vi "PipBoy_ReadFileConf.vi"(8 "error in (no error)":errorcluster) -> (0 "error out":errorcluster, 2 "FileConf":T1)   [LabVIEW 2014]
uses:
  ctls/PipBoy_FileConf.ctl
  <vilib>/Utility/config.llb/NI_LVConfig.lvlib
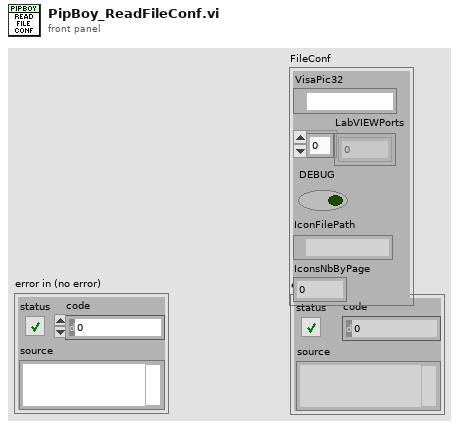
[diagram p1: front panel]
types:
  T1 = typedef "PipBoy_FileConf.ctl" = cluster{"VisaPic32":refnum<visa-resource-name>, "LabVIEWPorts":u16[], "DEBUG":bool, "IconFilePath":path, "IconsNbByPage":i32}
  T2 = typedef "NI_LVConfig.lvlib/Config Data RefNum.ctl" = refnum<k1>
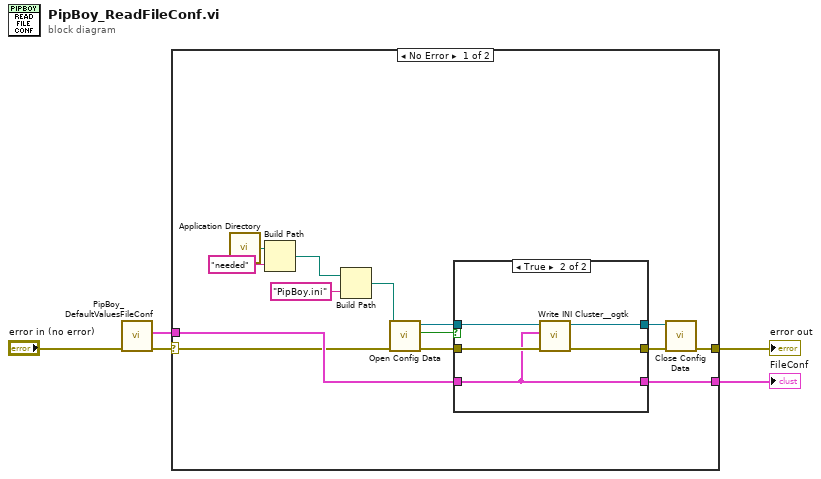
[diagram p0: block diagram]
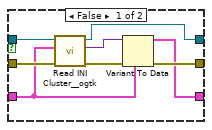
[diagram p2: hidden frame]
diagram:
  n1 = call "PipBoy_DefaultValuesFileConf.vi"("error in (no error)"="error in (no error)") -> ("error out"=w1:errorcluster, "FileConf"=w3:T1)  [unwired: 9 in]
  n2 = case shown="No Error" w1 {
    selector: w1 -> [w6 w34]
    tunnel: [w12 w34] -> w5
    tunnel: [w8 w33] -> w4
    tunnel: w3 -> [w7 w33]
    frame No Error {
      n3 = call <vilib>:"Application Directory.vi"() -> ("Application Directory"=w19:path)
      n4 = Build Path(base path=w19, name or relative path="needed") -> (appended path=w17:path)
      n5 = Build Path(base path=w17, name or relative path="PipBoy.ini") -> (appended path=w15:path)
      n6 = call <vilib>:"Open Config Data.vi"("error in (no error)"=w6, "configuration file path"=w15) -> ("error out"=w13:errorcluster, "file created?"=w14:bool, "refnum"=w9:T2)  [unwired: 7 in]
      n7 = case shown="True" w14 {
        tunnel: w13 -> [w27 w32]
        tunnel: [w25 w31] -> w11
        tunnel: w9 -> [w21 w29]
        tunnel: [w20 w28] -> w10
        tunnel: w7 -> [w23 w30]
        tunnel: [w22 w30] -> w8
        frame False {
          n8 = call <userlib>:"Read INI Cluster__ogtk.vi"("error in (no error)"=w27, "INI Fomatted Cluster Type"=w23, "refnum"=w21) -> ("error out"=w26:errorcluster, "INI Fomatted Cluster"=w24:variant, "dup refnum"=w20:T2)  [unwired: 4 in, 2 out]
          n9 = Variant To Data(error in=w26, type=w23, Variant=w24) -> (data=w22:T1, error out=w25:errorcluster)
        }
        frame True {
          n10 = call <userlib>:"Write INI Cluster__ogtk.vi"("error in (no error)"=w32, "INI Fomatted Cluster"=w30, "refnum"=w29) -> ("error out"=w31:errorcluster, "dup refnum"=w28:T2)  [unwired: 7 in]
        }
      }
      n11 = call <vilib>:"Close Config Data.vi"("error in (no error)"=w11, "refnum"=w10) -> ("error out"=w12:errorcluster)  [unwired: 8 in, 1 out]
    }
    frame Error {
    }
  }
  "error out" <- w5
  "FileConf" <- w4
